vi "_ConnectorPaneEditor_PAtternChange.vi"(8 "error in (no error)":errorcluster, 10 "NewVal":T1 items=["4800", "4803", "4806", "4801", "4802", "4805", "4830", "4804", "4807", "4831", "4832", "4810", "4808", "4809", "4811", "4812", "4816", "4823", "4824", "4817", "4818", "4825", "4819", "4813", "4820", "4826", "4821", "4827", "4828", "4822", "4814", "4829", "4815", "4833", "4834", "4835"], 11 "ConnectorPaneEditor in":refnum<class "_ConnectorPaneEditor.lvclass">) -> (0 "error out":errorcluster, 3 "ConnectorPaneEditor out":refnum<class "_ConnectorPaneEditor.lvclass">)   [LabVIEW 2014, in "_ConnectorPaneEditor.lvclass"]
uses:
  _ConnectorPaneEditor.lvclass
  Pattern.ctl
  _ConnectorPaneEditor.lvclass/_ConnectorPaneEditor.ctl
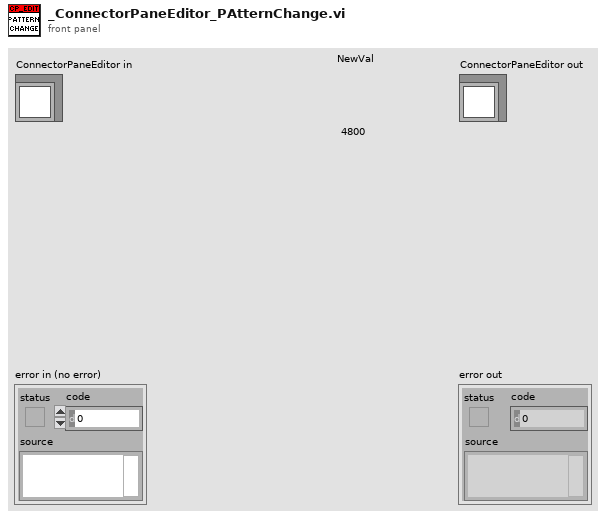
[diagram p1: front panel]
types:
  T1 = typedef "_ConnectorPaneEditor.lvclass/Pattern.ctl" = u16
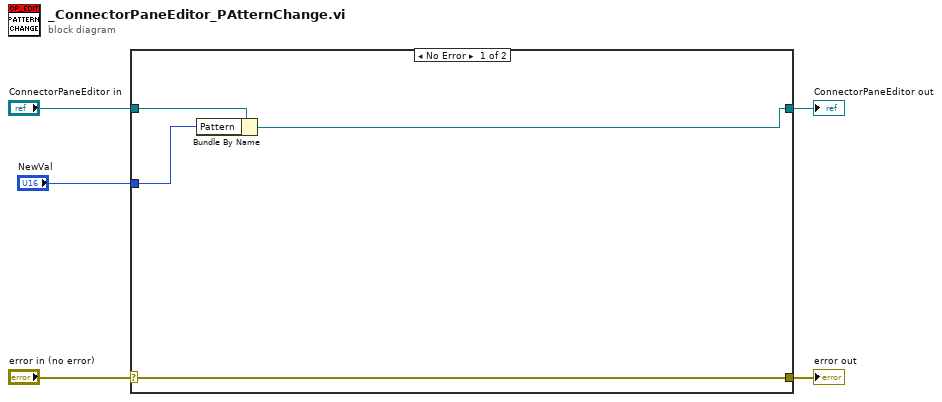
[diagram p0: block diagram]
diagram:
  n1 = case shown="No Error" "error in (no error)" {
    selector: "error in (no error)" -> [w9 w11]
    tunnel: [w9 w11] -> w4
    tunnel: [w6 w10] -> w2
    tunnel: "ConnectorPaneEditor in" -> [w8 w10]
    tunnel: "NewVal" -> [w7 _]
    frame No Error {
      n2 = Bundle By Name(cluster=w8, "Pattern"=w7) -> (w6:refnum<class "_ConnectorPaneEditor.lvclass">)
    }
    frame Error {
    }
  }
  "error out" <- w4
  "ConnectorPaneEditor out" <- w2
